vi "Read-Write_Check_Pos.vi"(5 "Simulate/Run":T1=enum."Run VI", 6 "!Offset Position by dx;dy;dz  Input":sgl[](array[numeric]), 7 "Position input":sgl[](array[numeric]), 8 "Mode":enum16{"Read", "Write"}(ring), 9 "Traverse Name":string="EnFlo Tunnel") -> (0 "!Offset Position by dx;dy;dz  Output":sgl[](array[numeric]), 1 "Position Output":sgl[](array[numeric]), 3 "Position Output with UW Offset":sgl[](array[numeric]))   [LabVIEW 2022 SP3]
uses:
  Controls/User_Specific_mode.ctl
  Globals/Constants_global.vi
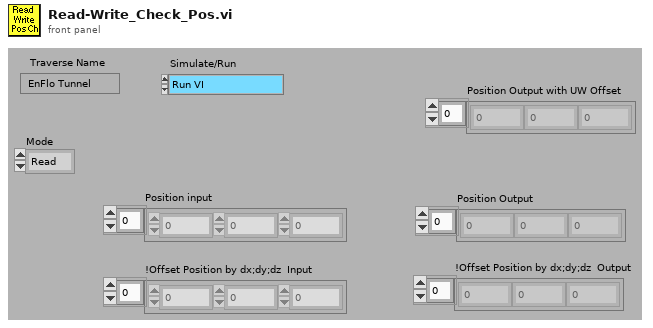
[diagram p1: front panel]
types:
  T1 = typedef "User_Specific_mode.ctl" = enum16{"Check VI only", "Run VI"}
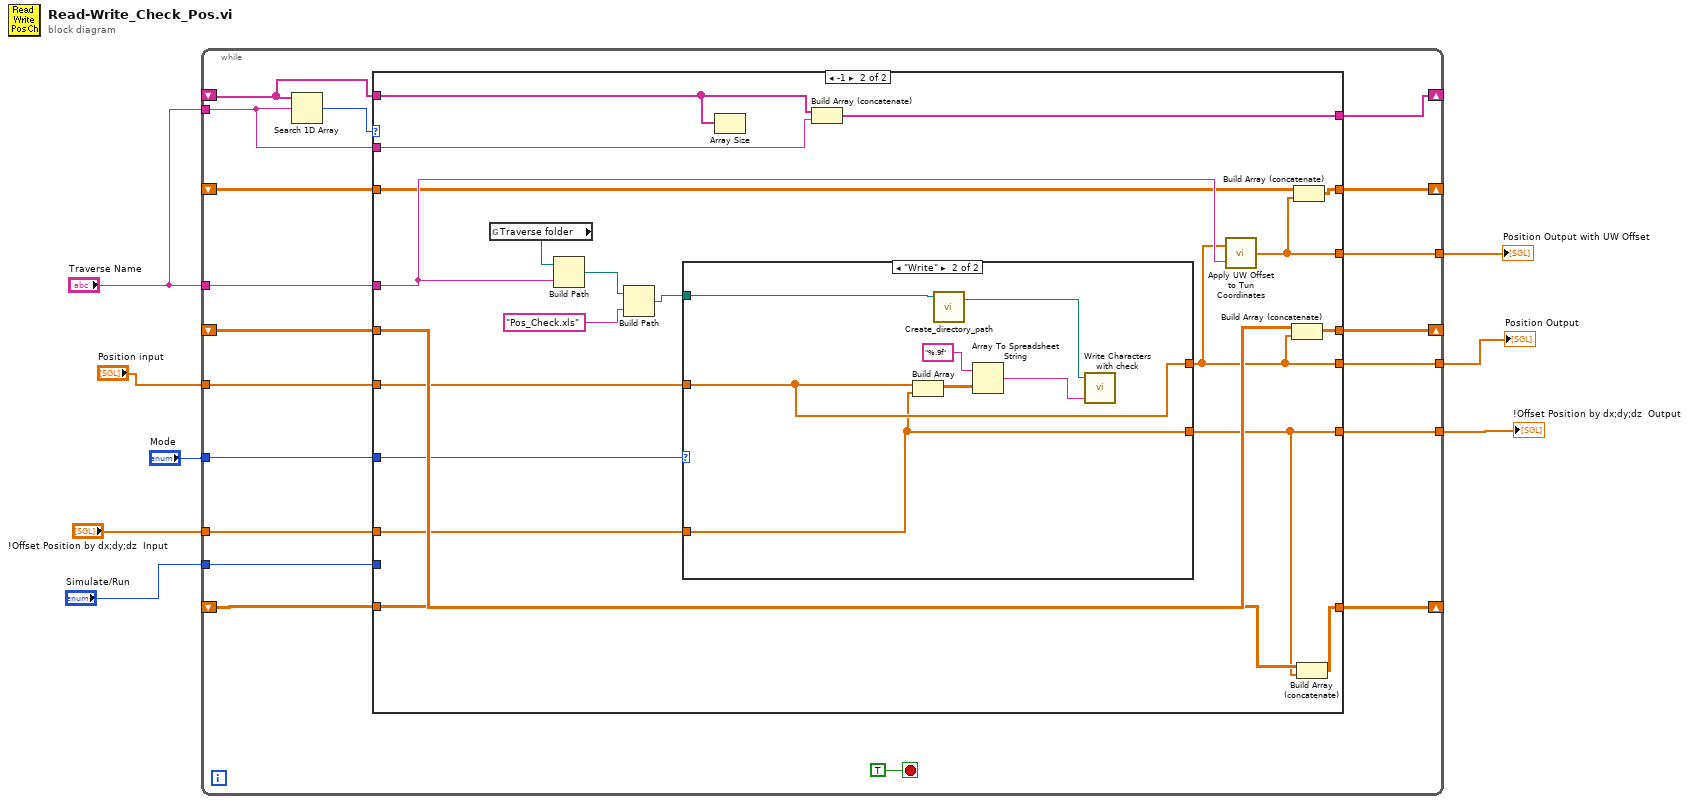
[diagram p0: block diagram]
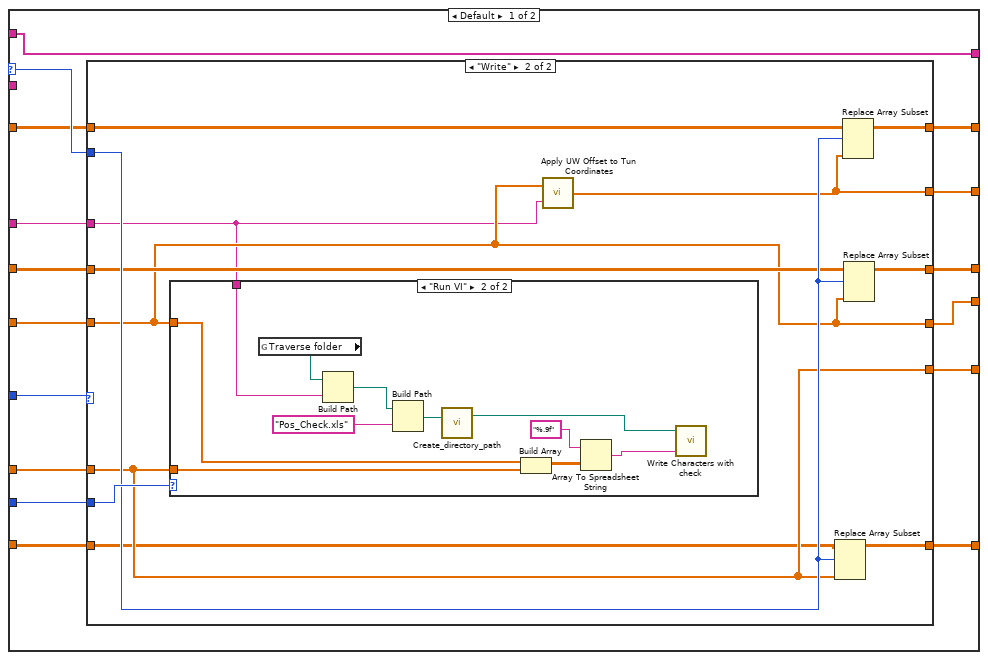
[diagram p2: hidden frame]
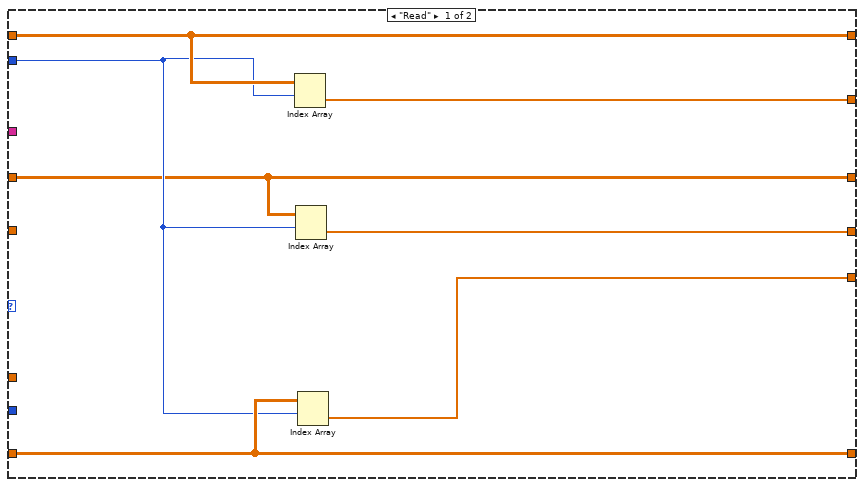
[diagram p3: hidden frame]
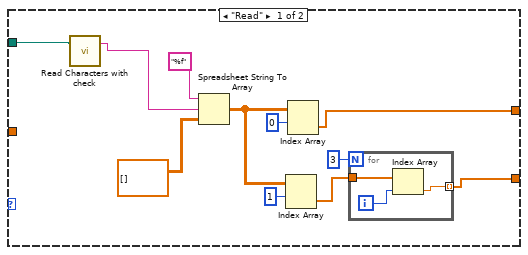
[diagram p5: hidden frame]
diagram:
  n1 = while {
    tunnel: "Traverse Name" -> [w27]
    tunnel: [w25] -> w8
    tunnel: [w24] -> w7
    shift-right: [w20] -> _
    shift-left: _ -> [w22]
    tunnel: "Traverse Name" -> [w21]
    tunnel: [w19] -> w5
    shift-right: [w17] -> _
    shift-left: _ -> [w18]
    shift-right: [w16] -> _
    shift-left: _ -> [w14]
    shift-right: [w15] -> _
    shift-left: _ -> [w13]
    tunnel: "Position input" -> [w12]
    tunnel: "Mode" -> [w11]
    tunnel: "!Offset Position by dx;dy;dz  Input" -> [w10]
    tunnel: "Simulate/Run" -> [w9]
    stop <- TRUE stop-if-true
    n2 = Search 1D Array(1D array=w22, element=w21) -> (index of element=w23:i32)  [unwired: 1 in]
    n3 = case shown="-1" w23 {
      selector: w23 -> [w41 _]
      tunnel: w27 -> [w28 w86]
      tunnel: [w40 w84] -> w25
      tunnel: [w33 w78] -> w24
      tunnel: w22 -> [w43 w87]
      tunnel: w21 -> [_ w89]
      tunnel: [w43 w88] -> w20
      tunnel: [w32 w77] -> w19
      tunnel: w18 -> [w39 w85]
      tunnel: [w38 w83] -> w17
      tunnel: [w36 w82] -> w16
      tunnel: [w34 w81] -> w15
      tunnel: w14 -> [w37 w80]
      tunnel: w13 -> [w35 w79]
      tunnel: w12 -> [w30 w76]
      tunnel: w11 -> [w42 w75]
      tunnel: w10 -> [w29 w74]
      tunnel: w9 -> [w31 _]
      frame Default {
        n4 = case shown="\"Write\"" w42 {
          tunnel: w41 -> [w47 w61]
          tunnel: [w50 w53] -> w40
          tunnel: w39 -> [w49 w55]
          tunnel: [w49 w60] -> w38
          tunnel: w37 -> [w46 w56]
          tunnel: [w46 w58] -> w36
          tunnel: w35 -> [w48 w51]
          tunnel: [w48 w59] -> w34
          tunnel: [w45 w57] -> w33
          tunnel: [w44 w54] -> w32
          tunnel: w31 -> [_ w62]
          tunnel: w30 -> [_ w54]
          tunnel: w29 -> [_ w57]
          tunnel: w28 -> [_ w52]
          frame "Read" {
            n5 = Index Array(array=w49, index (row)=w47) -> (element=w50:sgl[])  [unwired: 1 in]
            n6 = Index Array(array=w46, index (row)=w47) -> (element=w44:sgl[])  [unwired: 1 in]
            n7 = Index Array(array=w48, index (row)=w47) -> (element=w45:sgl[])  [unwired: 1 in]
          }
          frame "Write" {
            n8 = case shown="\"Run VI\"" w62 {
              tunnel: w54 -> [_ w67]
              tunnel: w57 -> [_ w66]
              tunnel: w52 -> [_ w65]
              frame "Check VI only" {
              }
              frame "Run VI" {
                n9 = global read "Constants_global.vi" "Traverse folder"() -> (w73:path)
                n10 = Build Path(base path=w73, name or relative path=w65) -> (appended path=w72:path)
                n11 = Build Path(base path=w72, name or relative path="Pos_Check.xls" ("string")) -> (appended path=w68:path)
                n12 = call "Create_directory_path.vi"("Path name"=w68) -> ("Path name Out"=w64:path)  [unwired: 2 in, 1 out]
                n13 = Build Array(w67, w66) -> (w69:sgl[][])
                n14 = Array To Spreadsheet String(array=w69, 3:"%.9f" ("format string")) -> (spreadsheet string=w63:string)  [unwired: 1 out]
                n15 = call "Write Characters with check.vi"("String to Write"=w63, "file (use dialog)"=w64) -> ()  [unwired: 2 in, 1 out]
              }
            }
            n16 = call "Apply UW Offset to Tun Coordinates.vi"("Traverse Name"=w52, "Tunnel Coordinates"=w54) -> ("UW Offset Applied"=w53:sgl[])
            n17 = Replace Array Subset(array=w51, new element=w57, index (row)=w61) -> (w59:sgl[][])  [unwired: 1 in]
            n18 = Replace Array Subset(array=w55, new element=w53, index (row)=w61) -> (w60:sgl[][])  [unwired: 1 in]
            n19 = Replace Array Subset(array=w56, new element=w54, index (row)=w61) -> (w58:sgl[][])  [unwired: 1 in]
          }
        }
      }
      frame -1 {
        n20 = global read "Constants_global.vi" "Traverse folder"() -> (w93:path)
        n21 = Build Path(base path=w93, name or relative path=w86) -> (appended path=w92:path)
        n22 = Build Path(base path=w92, name or relative path="Pos_Check.xls" ("string")) -> (appended path=w91:path)
        n23 = case shown="\"Write\"" w75 {
          tunnel: w91 -> [w95 w114]
          tunnel: [w97 w110] -> w78
          tunnel: [w96 w111] -> w77
          tunnel: w76 -> [_ w111]
          tunnel: w74 -> [_ w110]
          frame "Read" {
            n24 = call "Read Characters with check.vi"("file (use dialog)"=w95) -> ("Read String"=w94:string)  [unwired: 1 in, 1 out]
            n25 = Spreadsheet String To Array(format string="%f", spreadsheet string=w94, array type (2D Dbl)=sgl[][] []) -> (array=w102:sgl[][])  [unwired: 1 out]
            n26 = Index Array(array=w102, index (row)=1) -> (element=w100:sgl[])  [unwired: 1 in]
            n27 = Index Array(array=w102, index (row)=0) -> (element=w96:sgl[])  [unwired: 1 in]
            n28 = for {
              N: 3 -> [_]
              tunnel: w100 -> [w107]
              tunnel: [w105] -> w97 mode=indexing
              i -> [w106]
              n29 = Index Array(array=w107, index=w106) -> (element=w105:sgl)
            }
          }
          frame "Write" {
            n30 = Build Array(w111, w110) -> (w112:sgl[][])
            n31 = call "Create_directory_path.vi"("Path name"=w114) -> ("Path name Out"=w109:path)  [unwired: 2 in, 1 out]
            n32 = Array To Spreadsheet String(array=w112, 3:"%.9f" ("format string")) -> (spreadsheet string=w108:string)  [unwired: 1 out]
            n33 = call "Write Characters with check.vi"("String to Write"=w108, "file (use dialog)"=w109) -> ()  [unwired: 2 in, 1 out]
          }
        }
        n34 = Array Size(array=w87) -> ()  [unwired: 1 out]
        n35 = Build Array (concatenate)(w87, w89) -> (w88:string[])
        n36 = call "Apply UW Offset to Tun Coordinates.vi"("Traverse Name"=w86, "Tunnel Coordinates"=w77) -> ("UW Offset Applied"=w84:sgl[])
        n37 = Build Array (concatenate)(w80, w77) -> (w82:sgl[][])
        n38 = Build Array (concatenate)(w85, w84) -> (w83:sgl[][])
        n39 = Build Array (concatenate)(w79, w78) -> (w81:sgl[][])
      }
    }
  }
  "Position Output with UW Offset" <- w8
  "!Offset Position by dx;dy;dz  Output" <- w7
  "Position Output" <- w5
